vi "Periodic Tasks.vi"(8 "error in":errorcluster) -> ()   [LabVIEW 2020]
doc: "This VI runs in parallel to other tasks. It can contain as many user-defined periodic loops as you need. These can carry out PID or other sorts of timed response."
uses:
  <vilib>/Rock Robotics/WPI/Utilities/WPI_GetSetVariantRefNum.vi
  <vilib>/Rock Robotics/Network Tables/NT Read Number.vi
  Robot Global Data.vi
  <vilib>/Rock Robotics/Network Tables/NT Read Numeric Array.vi
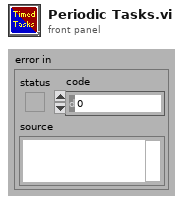
[diagram p1: front panel]
types:
  T1 = typedef "WPI_JoystickDevRef.ctl" = cluster{"Device":T2}
  T2 = typedef "WPI_JoystickDeviceEnum.ctl" = enum16{"USB 0", "USB 1", "USB 2", "USB 3", "USB 4", "USB 5"}
  T3 = typedef "WPI_RobotDriveDevRef.ctl" = cluster{"DevStatus":errorcluster, "Motors[]":T4[], "Square Inputs":bool, "Max Output":dbl}
  T4 = typedef "WPI_MotorControlDeviceRef.ctl" = cluster{"DeviceStatus":errorcluster, "Type":T5, "PWM":cluster{"PWM Channel":T6, "DeadBand":T7}, "CAN":cluster{"Device Number":u8, "SetOutput VI Ref":variant, "GetOutput VI Ref":variant, "Enable VI Ref":variant, "Disable VI Ref":variant, "Data":variant}, "Invert":bool, "DIO PWM":cluster{"PWM \"Enable\" Channel":T6, "DIOChannel":T8, "PWM Rate":dbl}}
  T5 = typedef "WPI_MotorControlType.ctl" = enum16{"PWM", "CAN", "DIO PWM"}
  T6 = typedef "FPGA_DIOPWMChannel.ctl" = enum8{"PWM 0", "PWM 1", "PWM 2", "PWM 3", "PWM 4", "PWM 5", "PWM 6", "PWM 7", "PWM 8", "PWM 9", "PWM MXP 0", "PWM MXP 1", "PWM MXP 2", "PWM MXP 3", "PWM MXP 4", "PWM MXP 5", "PWM MXP 6", "PWM MXP 7", "PWM MXP 8", "PWM MXP 9", "Invalid"}
  T7 = typedef "WPI_PWMDeadband.ctl" = cluster{"Name":string, "maxPositivePwm":i32, "minPositivePwm":i32, "centerPwm":i32, "maxNegativePwm":i32, "minNegativePwm":i32, "angularRange":u16}
  T8 = typedef "FPGA_DIOChannel.ctl" = enum8{"DIO 0", "DIO 1", "DIO 2", "DIO 3", "DIO 4", "DIO 5", "DIO 6", "DIO 7", "DIO 8", "DIO 9", "DIO MXP 0", "DIO MXP 1", "DIO MXP 2", "DIO MXP 3", "DIO MXP 4", "DIO MXP 5", "DIO MXP 6", "DIO MXP 7", "DIO MXP 8", "DIO MXP 9", "DIO MXP 10", "DIO MXP 11", "DIO MXP 12", "DIO MXP 13", "DIO MXP 14", "DIO MXP 15", "SPI Port CS1", "SPI Port CS2", "SPI Port CS3", "SPI Port MISO", "SPI Port MOSI", "Invalid"}
  T9 = cluster{"JoystickDevRef":T1, "RobotDriveDevRef":T3}
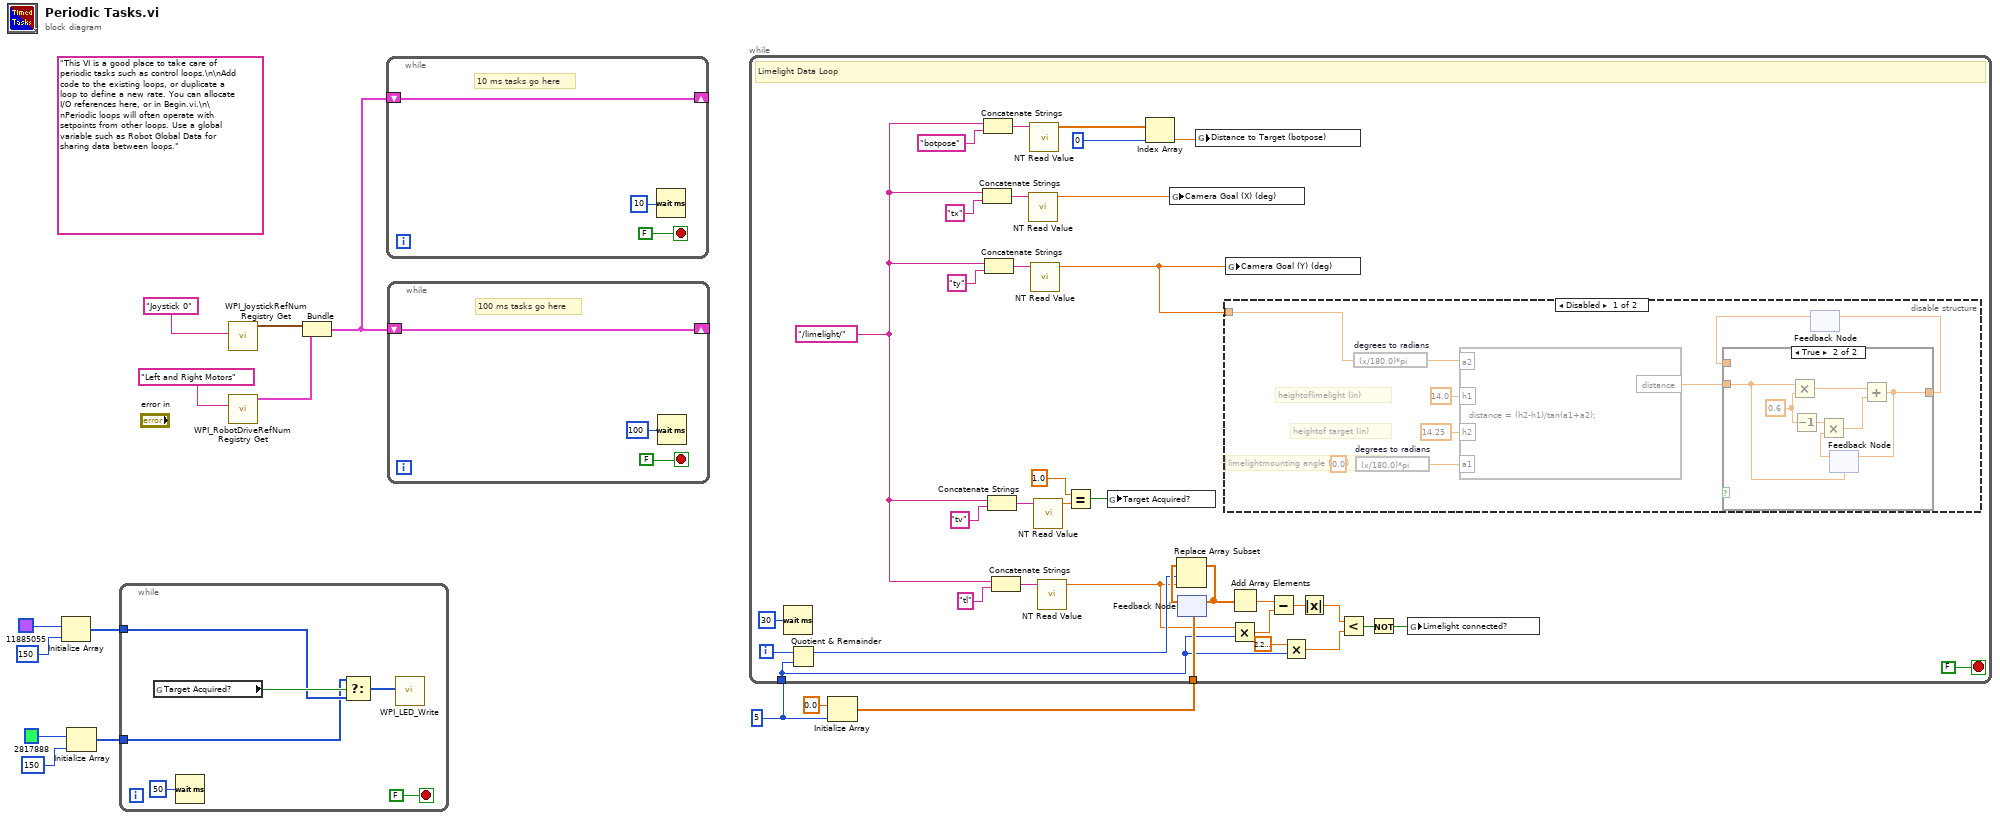
[diagram p0: block diagram]
diagram:
  w8 = 5
  (unwired) "This VI is a good place to take care of periodic tasks such as control loops.\n\nAdd code to the existing loops, or duplicate a loop to define a new rate. You can allocate I/O references here, or in Begin.vi.\n\nPeriodic loops will often operate with setpoints from other loops. Use a global variable such as Robot Global Data for sharing data between loops."
  n1 = Initialize Array(u32 11885055, 150 ("dimension size")) -> (w4:u32[])
  n2 = Initialize Array(u32 2817888, 150 ("dimension size")) -> (w1:u32[])
  n3 = while {
    tunnel: w4 -> [w16]
    tunnel: w1 -> [w15]
    stop <- FALSE stop-if-true
    n4 = global read "Robot Global Data.vi" "Target Acquired?"() -> (w17:bool)
    n5 = Wait (ms)(milliseconds to wait=u32 50) -> ()  [unwired: 1 out]
    n6 = Select(t=w15, s=w17, f=w16) -> (s? t:f=w18:u32[])
    n7 = call <vilib>:"WPI_LED_Write.vi"("Color Array"=w18) -> ()  [unwired: 10 in, 1 out]
  }
  n8 = call <vilib>:"WPI_JoystickRefNum Registry Get.vi"("refnum name"="Joystick 0") -> ("JoystickDevRef"=w12:T1)  [unwired: 1 in, 9 out]
  n9 = call <vilib>:"WPI_RobotDriveRefNum Registry Get.vi"("refnum name"="Left and Right Motors") -> ("RobotDriveDevRef"=w11:T3)  [unwired: 1 in, 9 out]
  n10 = Bundle("JoystickDevRef"=w12, "RobotDriveDevRef"=w11) -> (w10:T9)  [unwired: 1 out]
  n11 = while {
    shift-right: [w21] -> _
    shift-left: w10 -> [w21]
    stop <- FALSE stop-if-true
    # "10 ms tasks go here"
    n12 = Wait (ms)(milliseconds to wait=u32 10) -> ()  [unwired: 1 out]
  }
  n13 = while {
    shift-right: [w24] -> _
    shift-left: w10 -> [w24]
    stop <- FALSE stop-if-true
    # "100 ms tasks go here"
    n14 = Wait (ms)(milliseconds to wait=u32 100) -> ()  [unwired: 1 out]
  }
  n15 = Initialize Array(0.0 ("element"), w8) -> (w7:dbl[])
  n16 = while {
    tunnel: w8 -> [w44]
    tunnel: w7 -> [w50]
    i -> [w53]
    stop <- FALSE stop-if-true
    w34 = "/limelight/"
    # "Limelight Data Loop"
    n17 = Wait (ms)(milliseconds to wait=u32 30) -> ()  [unwired: 1 out]
    n18 = Quotient & Remainder(x=w53, y=w44) -> (x-y*floor(x/y)=w51:i32)  [unwired: 1 out]
    n19 = Concatenate Strings(w34, "tx" ("string")) -> (w60:string)
    n20 = Concatenate Strings(w34, "botpose" ("string")) -> (w35:string)
    n21 = Concatenate Strings(w34, "ty" ("string")) -> (w58:string)
    n22 = Concatenate Strings(w34, "tv" ("string")) -> (w56:string)
    n23 = Concatenate Strings(w34, "tl" ("string")) -> (w54:string)
    n24 = call-poly <vilib>:"NT Read Value.vi"("name"=w60) -> ("value"=w30:dbl)  [unwired: 8 in, 2 out]
    n25 = call-poly <vilib>:"NT Read Value.vi"("name"=w35) -> ("value"=w33:dbl[])  [unwired: 8 in, 2 out]
    n26 = call-poly <vilib>:"NT Read Value.vi"("name"=w58) -> ("value"=w29:dbl)  [unwired: 8 in, 2 out]
    n27 = call-poly <vilib>:"NT Read Value.vi"("name"=w56) -> ("value"=w38:dbl)  [unwired: 8 in, 2 out]
    n28 = call-poly <vilib>:"NT Read Value.vi"("name"=w54) -> ("value"=w46:dbl)  [unwired: 8 in, 2 out]
    n29 = Equal?(x=1.0, y=w38) -> (x = y?=w28:bool)
    n30 = global write "Robot Global Data.vi" "Target Acquired?"(w28) -> ()
    n31 = Index Array(array=w33, index=0) -> (element=w31:dbl)
    n32 = global write "Robot Global Data.vi" "Camera Goal (X) (deg)"(w30) -> ()
    n33 = feedback #1(w50) -> (w52:dbl[])
    n34 = Replace Array Subset(array=w52, new element=w46, index=w51) -> (w49:dbl[])
    n35 = feedback-in #1(w49) -> ()
    n36 = global write "Robot Global Data.vi" "Distance to Target (botpose)"(w31) -> ()
    n37 = disable-structure shown="Disabled" {
      disable-tunnel: w29 -> [w63 _]
      frame Disabled {
        # "limelightmounting angle (deg)"
        # "heightof target (in)"
        # "heightoflimelight (in)"
        n38 = expression code="(x/180.0)*pi" "degrees to radians"(w63) -> (w72:dbl)
        n39 = expression code="(x/180.0)*pi" "degrees to radians"(0.0 ("value")) -> (w69:dbl)
        n40 = formula code="distance = (h2-h1)/tan(a1+a2);"("a2"=w72, "a1"=w69, "h1"=14.0 ("input variable"), "h2"=14.25 ("input variable")) -> ("distance"=w67:dbl)
        n41 = feedback #2() -> (w66:dbl)  [unwired: 1 in]
        n42 = case shown="True" w64 {
          tunnel: w67 -> [_ w78]
          tunnel: [w73 w74] -> w65
          tunnel: w66 -> [w73 _]
          frame False {
          }
          frame True {
            w79 = 0.6
            n43 = Multiply(x=w78, y=w79) -> (x*y=w76:dbl)
            n44 = Decrement(x=w79) -> (x-1=w80:dbl)
            n45 = feedback #3(w78) -> (w77:dbl)
            n46 = Multiply(x=w80, y=w77) -> (x*y=w75:dbl)
            n47 = Add(x=w76, y=w75) -> (x+y=w74:dbl)
            n48 = feedback-in #3(w74) -> ()
          }
        }
        n49 = feedback-in #2(w65) -> ()
      }
      frame Enabled {
      }
    }
    n50 = global write "Robot Global Data.vi" "Camera Goal (Y) (deg)"(w29) -> ()
    n51 = Multiply(x=w46, y=w44) -> (x*y=w47:dbl)
    n52 = Add Array Elements(numeric array=w49) -> (sum=w48:dbl)
    n53 = Subtract(x=w48, y=w47) -> (x-y=w43:dbl)
    n54 = Multiply(x=2.220446049250313e-16, y=w44) -> (x*y=w41:dbl)
    n55 = Absolute Value(x=w43) -> (abs(x)=w42:dbl)
    n56 = Less?(x=w42, y=w41) -> (x < y?=w40:bool)
    n57 = Not(x=w40) -> (.not. x?=w27:bool)
    n58 = global write "Robot Global Data.vi" "Limelight connected?"(w27) -> ()
  }
